vi "Set ListSelection.lvclass.vi"(8 "error in (no error)":errorcluster, 10 "Admin_Actor.lvlib:ListSelection.lvclass":refnum<class "ListSelection.lvclass">, 11 "ExcuseNotesHandler in":refnum<class "ExcuseNotesHandler.lvclass">) -> (0 "error out":errorcluster, 3 "ExcuseNotesHandler out":refnum<class "ExcuseNotesHandler.lvclass">)   [LabVIEW 2015, in "ExcuseNotesHandler.lvclass"]
uses:
  ExcuseNotesHandler.lvclass
  Models/ListSelection/ListSelection.lvclass
  ExcuseNotesHandler.lvclass/ExcuseNotesHandler.ctl
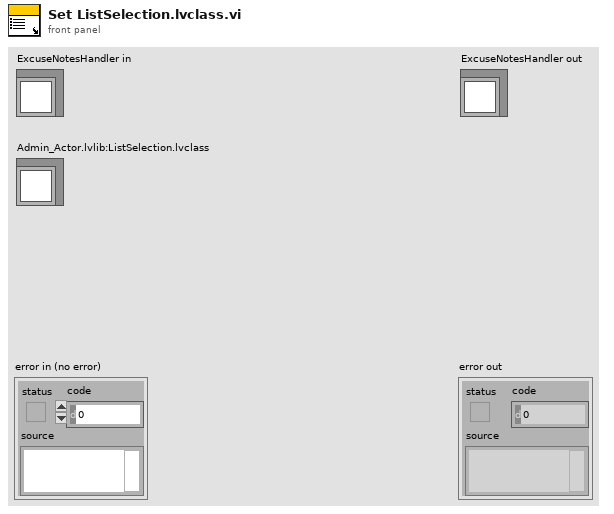
[diagram p1: front panel]
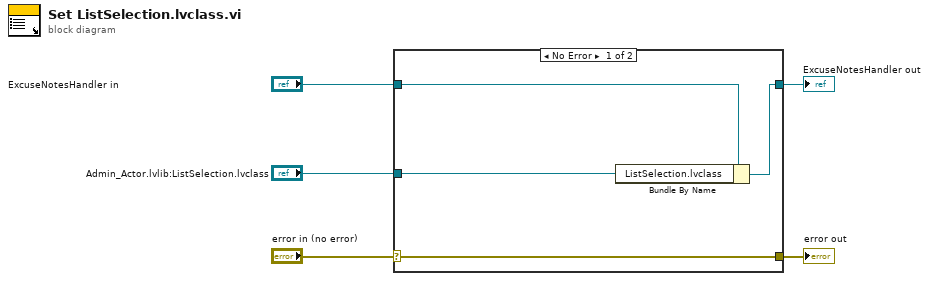
[diagram p0: block diagram]
diagram:
  n1 = case shown="No Error" "error in (no error)" {
    selector: "error in (no error)" -> [w9 w10]
    tunnel: [w9 w10] -> w4
    tunnel: [w7 w11] -> w2
    tunnel: "ExcuseNotesHandler in" -> [w8 w11]
    tunnel: "Admin_Actor.lvlib:ListSelection.lvclass" -> [w6 _]
    frame No Error {
      n2 = Bundle By Name(cluster=w8, "ListSelection.lvclass"=w6) -> (w7:refnum<class "ExcuseNotesHandler.lvclass">)
    }
    frame Error {
    }
  }
  "error out" <- w4
  "ExcuseNotesHandler out" <- w2
